vi "Autonomous Joystick Emulation.vi"() -> ()   [LabVIEW 2012]
panel:
  in  "Joy Y Command":dbl
  in  "Joy X Command":dbl
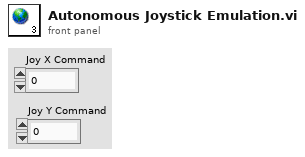
[diagram p1: front panel]
diagram:
